vi "Get Desired Positon.vi"(8 "error in (no error)":errorcluster, 11 "FINE SIM Motion Axis":refnum<class "FINE SIM Motion Axis.lvclass">) -> (0 "error out":errorcluster, 2 "Raw Current Position":dbl, 3 "FINE SIM Motion Axis":refnum<class "FINE SIM Motion Axis.lvclass">)   [LabVIEW 2022 SP3, in "FINE SIM Motion Axis.lvclass"]
uses:
  FINE SIM Motion Axis.lvclass
  FINE SIM Motion Axis.lvclass/FINE SIM Motion Axis.ctl
  Accessors/Read Sim Axis Data.vi
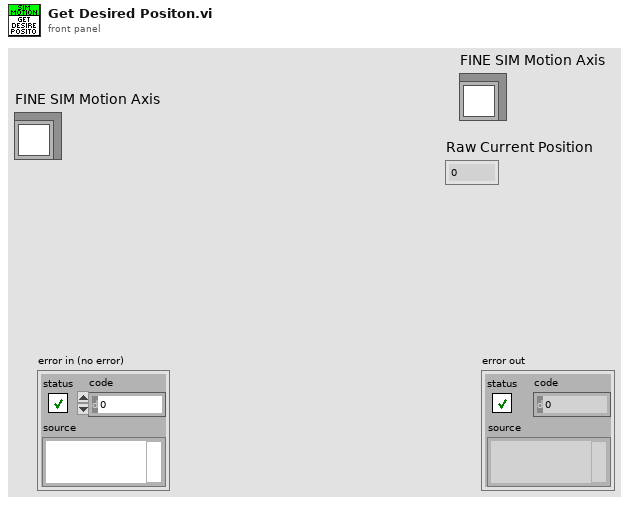
[diagram p1: front panel]
types:
  T1 = typedef "FINE SIM Motion Axis.lvclass/Axis Data.ctl" = cluster{"Axis Parameters":T2, "Axis Settings":T4, "Time Stamp":timestamp}
  T2 = typedef "FINE SIM Motion Axis.lvclass/Axis Parameters.ctl" = cluster{"Moving":bool, "Homed":bool, "Desired Position":dbl, "Current Positon":dbl, "Current Speed":dbl, "Home Status":T3}
  T3 = typedef "FINE SIM Motion Axis.lvclass/Homing Status.ctl" = enum16{"Idle", "Inital Home Motion", "Final Home Motion", "Done Homing"}
  T4 = typedef "FINE SIM Motion Axis.lvclass/Axis Settings.ctl" = cluster{"Speed":dbl, "Acceleration":dbl}
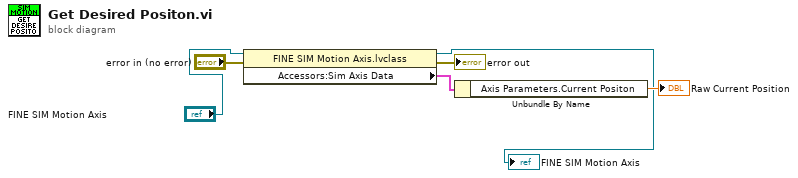
[diagram p0: block diagram]
diagram:
  n1 = property class="FINE SIM Motion Axis.lvclass"(reference="FINE SIM Motion Axis", error in="error in (no error)") -> (reference out=→"FINE SIM Motion Axis":refnum<class "FINE SIM Motion Axis.lvclass">, error out=→"error out":errorcluster, "Accessors:Sim Axis Data"=w3:T1)
  n2 = Unbundle By Name(w3) -> ("Axis Parameters.Current Positon"=→"Raw Current Position":dbl)
